vi "test1-LocalExternalStatusRegistration.vi"(8 "error in (no error)":errorcluster, 11 "TestCase in":refnum<class "testcase-CSMBroadcast.lvclass">) -> (0 "error out":errorcluster, 3 "TestCase out":refnum<class "testcase-CSMBroadcast.lvclass">)   [LabVIEW 2017, in "testcase-CSMBroadcast.lvclass"]
uses:
  testcase-CSMBroadcast.lvclass
  0b17d103-e67b-41be-a9eb-a2ee1311ff1f.vi
  5999693e-4f8a-4b34-ae87-f34dff5771be.vi
  de2dcf32-e0f3-4ce3-ae15-c78c2a65fbc0.vi
  52a2a10a-a04b-4bad-8df4-e1eb944f47cc.vi
  826f03dd-b4b5-4c6b-9085-8edf6da4f43b.vi
  src/user.lib/_NEVSTOP/Communicable State Machine(CSM)/AdvanceAPI/CSM - Revert Arguments-Safe String.vi
  src/user.lib/_NEVSTOP/Communicable State Machine(CSM)/_Shared/Trim Single-line Text.vi
  src/user.lib/_NEVSTOP/Communicable State Machine(CSM)/AdvanceAPI/CSM - Make String Arguments Safe.vi
  src/user.lib/_NEVSTOP/Communicable State Machine(CSM)/AdvanceAPI/CSM - Break Down Multiple States String.vi
  src/user.lib/_NEVSTOP/Communicable State Machine(CSM)/AdvanceAPI/CSM - Keywords.vi
  src/user.lib/_NEVSTOP/Communicable State Machine(CSM)/_Polymophic/CSM - Replace Marks in Messages.vi
  src/user.lib/_NEVSTOP/Communicable State Machine(CSM)/AdvanceAPI/CSM - Get Module Attribute.vi
  <vilib>/addons/_JKI Toolkits/VI Tester/TestCase.llb/TestCase.lvclass
  src/user.lib/_NEVSTOP/Communicable State Machine(CSM)/Communicable State Machine.lvlib
  C:/Program Files (x86)/National Instruments/LabVIEW 2017/vi.lib/addons/_JKI Toolkits/VI Tester/TestCase.llb/TestCase.lvclass
panel:
  out "One-Shot Unregistrations":string
  out "One-Shot Registrations":string
  out "LoopCount 2":i32
  out "State History":string
  out "LoopCount":i32
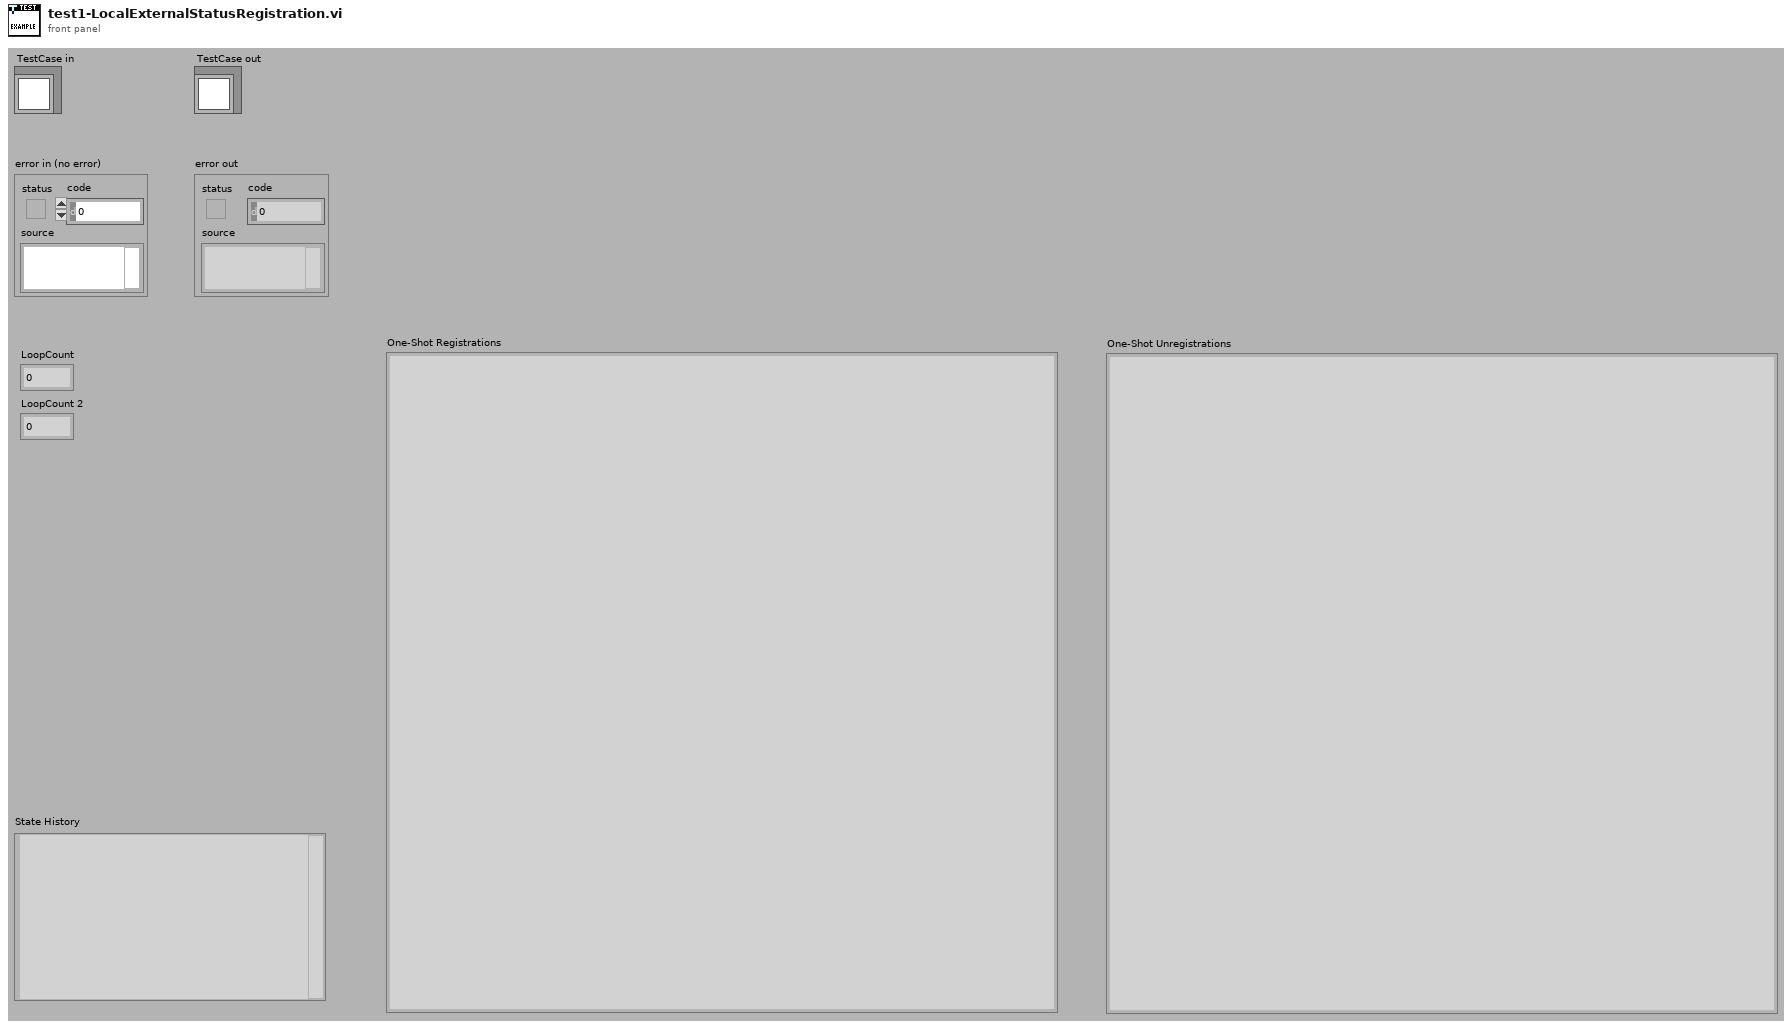
[diagram p1: front panel]
types:
  T1 = enum32{"Invalid", "Standard", "Closed", "Hidden", "Minimized", "Maximized"}
  T2 = enum32{"invalid app kind", "Development System", "Run Time System", "Student Edition", "Embedded LabVIEW", "Evaluation", "Custom"}
  T3 = typedef "Communicable State Machine.lvlib/_CSM_Response Source Message.ctl" = cluster{"‘State":string, "’Arguments":string, "’Error":errorcluster}
  T4 = cluster{"Current VI Reference":refnum<vi>, "Close Panel on Exit?":bool}
  T5 = cluster{"Core":cluster{"Current VI Reference":refnum<vi>, "Close Panel on Exit?":bool}, "Your Boolean data":bool, "Your string data":string}
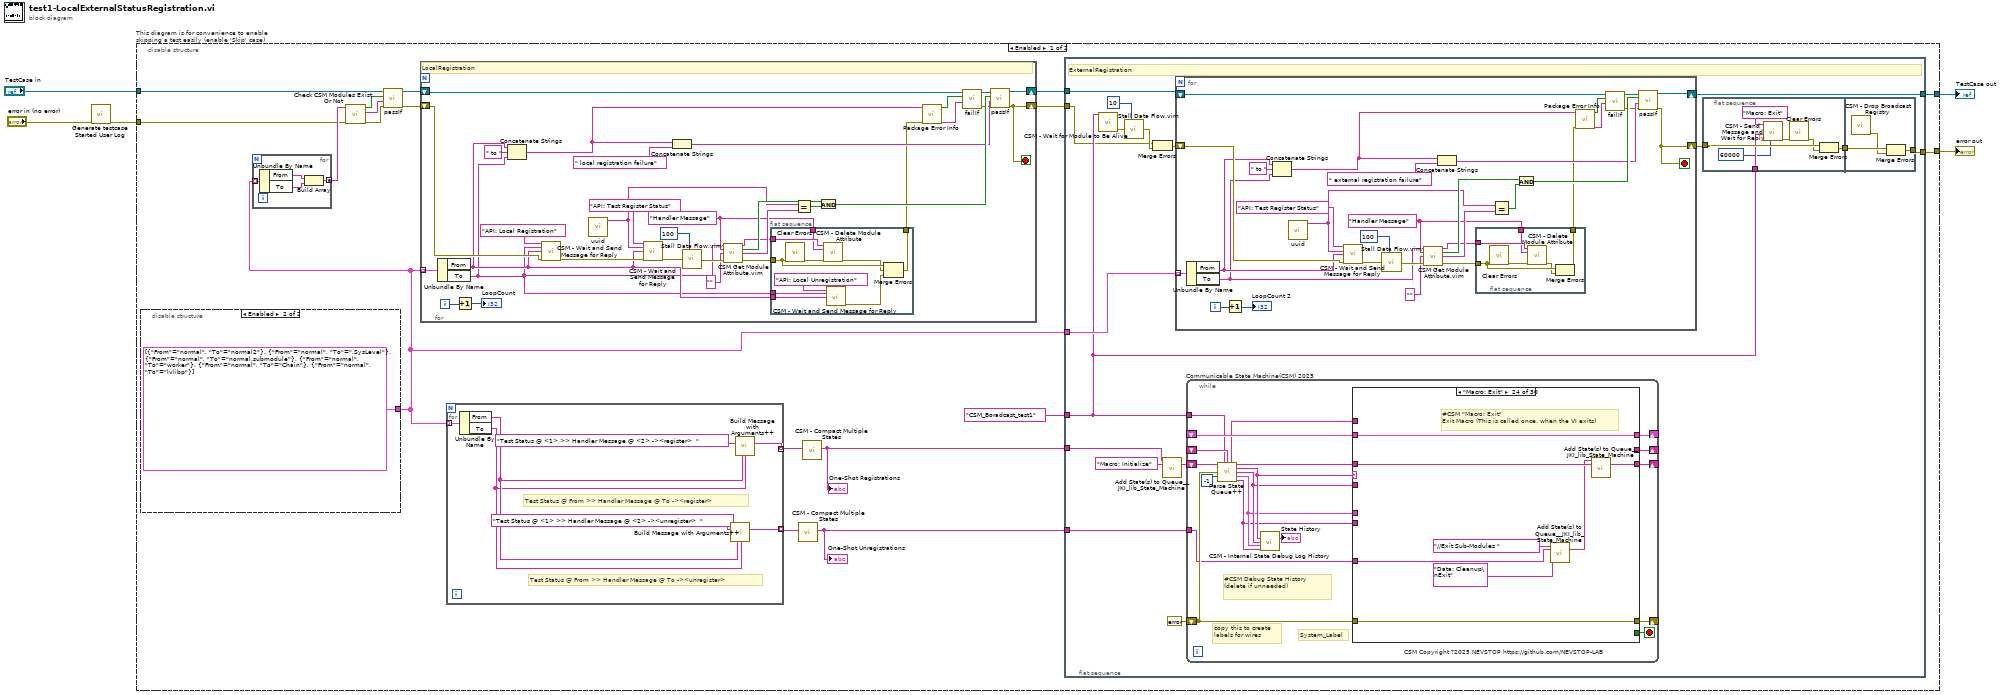
[diagram p0: block diagram]
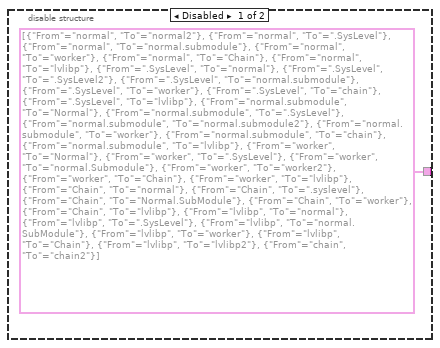
[diagram p2: hidden frame]
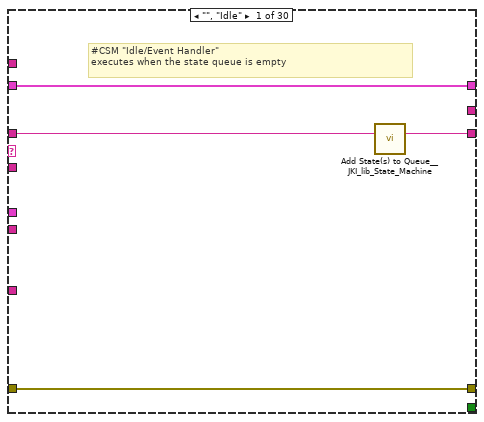
[diagram p3: hidden frame]
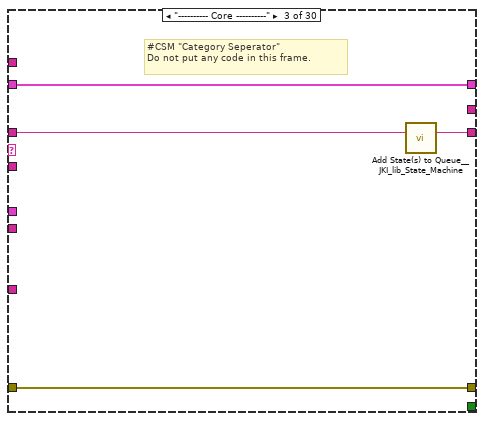
[diagram p5: hidden frame]
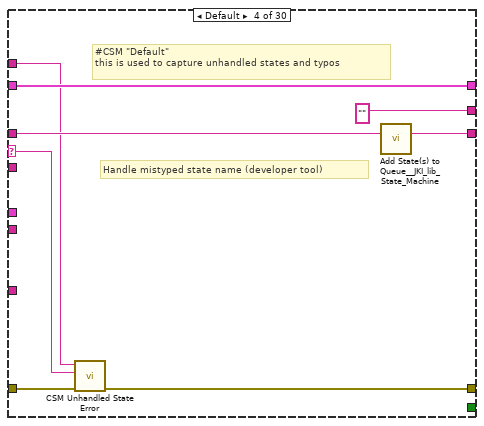
[diagram p6: hidden frame]
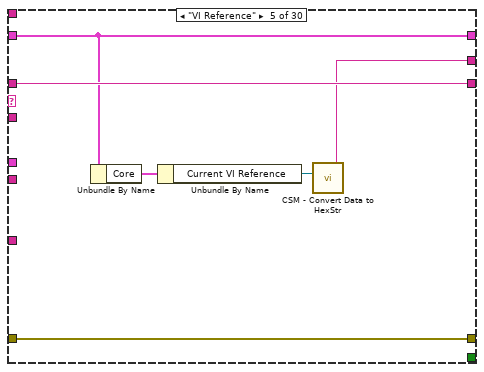
[diagram p7: hidden frame]
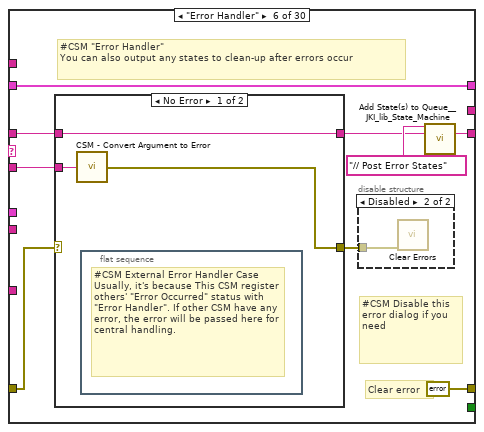
[diagram p8: hidden frame]
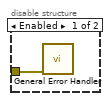
[diagram p9: hidden frame]
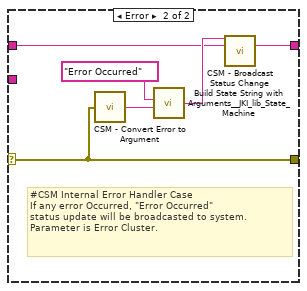
[diagram p10: hidden frame]
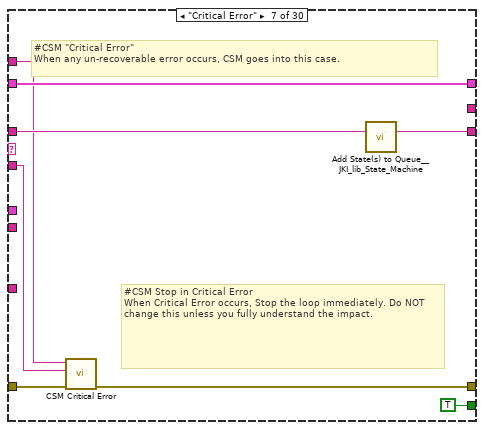
[diagram p11: hidden frame]
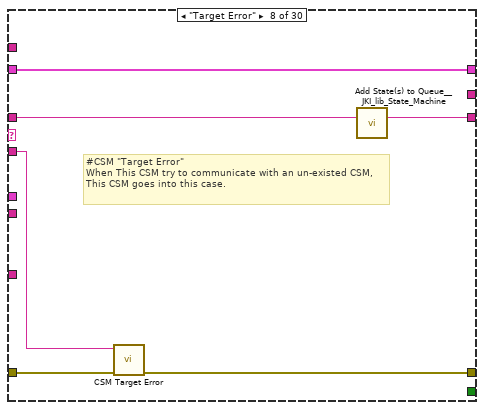
[diagram p12: hidden frame]
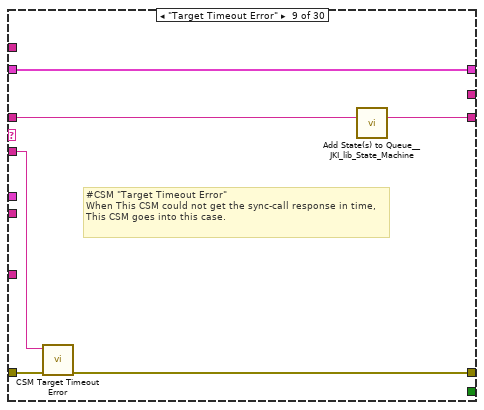
[diagram p13: hidden frame]
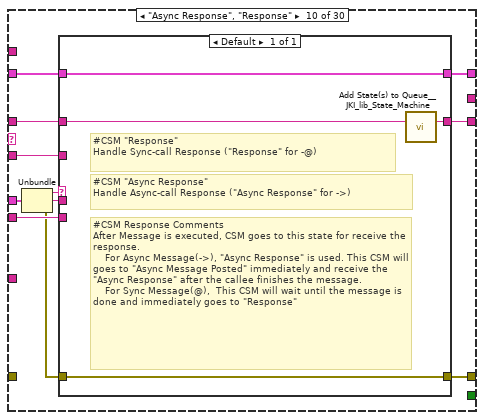
[diagram p14: hidden frame]
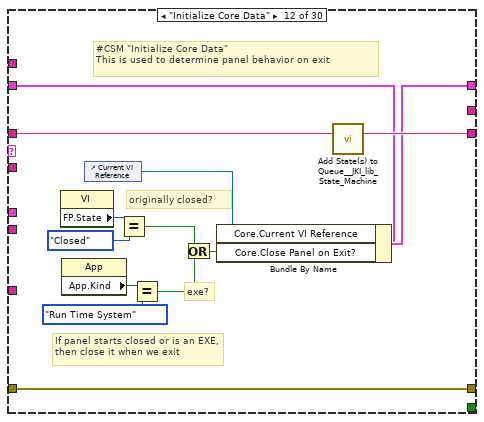
[diagram p16: hidden frame]
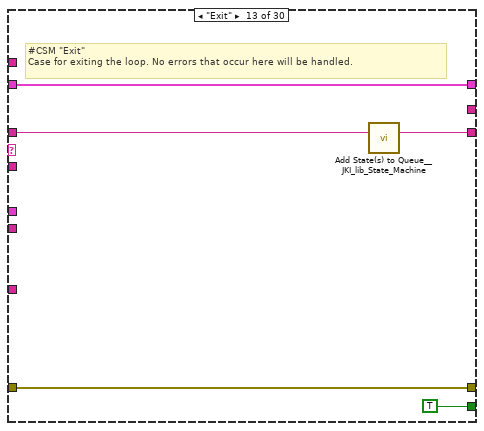
[diagram p17: hidden frame]
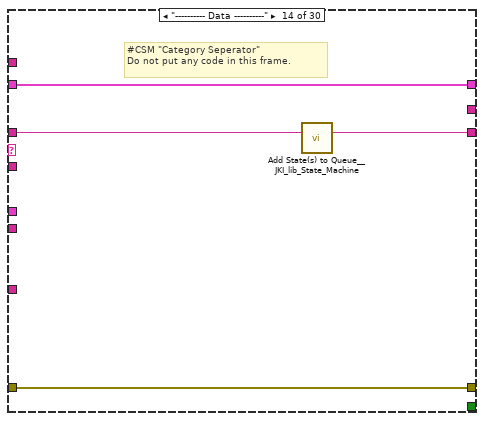
[diagram p18: hidden frame]
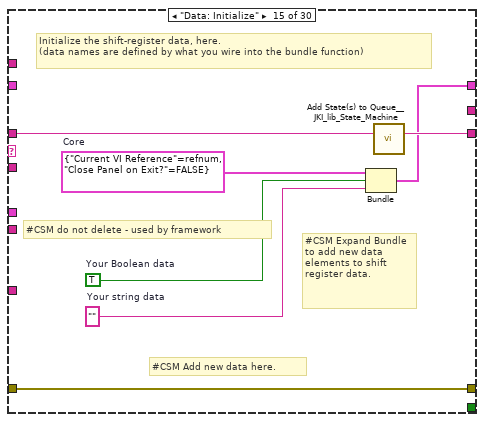
[diagram p19: hidden frame]
diagram:
  n1 = call "Generate testcase Started User Log.vi"("Error In"="error in (no error)") -> ("error out"=w1:errorcluster)  [unwired: 10 in]
  n2 = disable-structure "This diagram is for convenience to enable skipping a test easily (enable 'Skip' case)" shown="Enabled" {
    disable-tunnel: "TestCase in" -> [w11 w424]
    disable-tunnel: [w22 w422] -> w2
    disable-tunnel: [w16 w423] -> w4
    disable-tunnel: w1 -> [w9 w421]
    frame Enabled {
      n3 = disable-structure shown="Enabled" {
        disable-tunnel: [cluster{"From":string, "To":string}[] [{"From"="normal", "To"="normal2"}, {"From"="normal", "To"=".SysLevel"}, {"From"="normal", "To"="normal.submodule"}, {"From"="normal", "To"="worker"}, {"From"="normal", "To"="Chain"}, {"From"="normal", "To"="lvlibp"}, {"From"=".SysLevel", "To"="normal"}, {"From"=".SysLevel", "To"=".SysLevel2"}, {"From"=".SysLevel", "To"="normal.submodule"}, {"From"=".SysLevel", "To"="worker"}, {"From"=".SysLevel", "To"="chain"}, {"From"=".SysLevel", "To"="lvlibp"}, {"From"="normal.submodule", "To"="Normal"}, {"From"="normal.submodule", "To"=".SysLevel"}, {"From"="normal.submodule", "To"="normal.submodule2"}, {"From"="normal.submodule", "To"="worker"}, {"From"="normal.submodule", "To"="chain"}, {"From"="normal.submodule", "To"="lvlibp"}, {"From"="worker", "To"="Normal"}, {"From"="worker", "To"=".SysLevel"}, {"From"="worker", "To"="normal.Submodule"}, {"From"="worker", "To"="worker2"}, {"From"="worker", "To"="Chain"}, {"From"="worker", "To"="lvlibp"}, {"From"="Chain", "To"="normal"}, {"From"="Chain", "To"=".syslevel"}, {"From"="Chain", "To"="Normal.SubModule"}, {"From"="Chain", "To"="worker"}, {"From"="Chain", "To"="lvlibp"}, {"From"="lvlibp", "To"="normal"}, {"From"="lvlibp", "To"=".SysLevel"}, {"From"="lvlibp", "To"="normal.SubModule"}, {"From"="lvlibp", "To"="worker"}, {"From"="lvlibp", "To"="Chain"}, {"From"="lvlibp", "To"="lvlibp2"}, {"From"="chain", "To"="chain2"}] cluster{"From":string, "To":string}[] [{"From"="normal", "To"="normal2"}, {"From"="normal", "To"=".SysLevel"}, {"From"="normal", "To"="normal.submodule"}, {"From"="normal", "To"="worker"}, {"From"="normal", "To"="Chain"}, {"From"="normal", "To"="lvlibp"}]] -> w6
        frame Disabled {
        }
        frame Enabled {
        }
      }
      n4 = for {
        tunnel: w6 -> [w29] mode=indexing
        tunnel: [w26] -> w14 mode=concatenating
        n5 = Unbundle By Name(w29) -> ("From"=w28:string, "To"=w27:string)
        n6 = Build Array(w28, w27) -> (w26:string[])
      }
      n7 = call "Check CSM Modules Exist Or Not.vi"("error in"=w9, "CSM names in"=w14) -> ("error out"=w12:errorcluster, "Debug string"=w13:string, "All Modules Exist?"=w15:bool)  [unwired: 7 in]
      n8 = call-dynamic "passIf.vi"("error in (no error)"=w12, "message (\"\")"=w13, "pass"=w15, "TestCase in"=w11) -> ("error out"=w8:errorcluster, "TestCase out"=w10:refnum<class "testcase-CSMBroadcast.lvclass">)  [unwired: 6 in]
      n9 = for {
        shift-right: [w42] -> w21
        shift-left: w8 -> [w43]
        shift-right: [w49] -> w23
        shift-left: w10 -> [w34]
        tunnel: w6 -> [w60] mode=indexing
        i -> [w62]
        stop <- w42 stop-if-true
        w44 = "Handler Message" ("To")
        # "LocalRegistration"
        n10 = Unbundle By Name(w60) -> ("From"=w40:string, "To"=w39:string)
        n11 = Increment(x=w62) -> (x+1=→"LoopCount":i32)
        n12 = Concatenate Strings(w40, " to " ("string"), w39) -> (w30:string)
        n13 = call "CSM - Wait and Send Message for Reply.vi"("State"="API: Local Registration", "Arguments (\"\")"=w39, "Target Module"=w40, "Error In (No Error)"=w43) -> ("error out"=w57:errorcluster)  [unwired: 8 in, 3 out]
        n14 = call "uuid.vi"() -> ("UUID"=w51:string)  [unwired: 11 in]
        n15 = call "CSM - Wait and Send Message for Reply.vi"("State"="API: Test Register Status", "Arguments (\"\")"=w51, "Target Module"=w40, "Error In (No Error)"=w57) -> ("error out"=w56:errorcluster)  [unwired: 8 in, 3 out]
        n16 = Concatenate Strings(w30, " local registration failure" ("string")) -> (w37:string)
        n17 = call "Stall Data Flow.vim"("value in"=w56, "milliseconds to wait"=u32 100) -> ("value out"=w54:errorcluster)  [unwired: 1 out]
        n18 = call "CSM Get Module Attribute.vim"("CSM Name"=w39, "Attribute"=w44, "Default Value (Empty Variant)"="", "Error In"=w54) -> ("CSM Name (Dup)"=w45:string, "Found"=w53:bool, "Value"=w50:string, "error out"=w46:errorcluster)  [unwired: 7 in, 1 out]
        n19 = flat-sequence {
          tunnel: w46 -> [w66]
          tunnel: w45 -> [w71]
          tunnel: w44 -> [w70]
          tunnel: w39 -> [w68]
          tunnel: w40 -> [w67]
          tunnel: [w63] -> w31
          frame #0 {
            n20 = call <vilib>:"Clear Errors.vi"("error in (no error)"=w66) -> ("error out"=w72:errorcluster)  [unwired: 5 in, 1 out]
            n21 = call "CSM - Delete Module Attribute.vi"("CSM Name"=w71, "Attribute"=w70, "Error In"=w72) -> ("error out"=w65:errorcluster)  [unwired: 9 in, 3 out]
            n22 = call "CSM - Wait and Send Message for Reply.vi"("State"="API: Local Unregistration", "Arguments (\"\")"=w68, "Target Module"=w67) -> ("error out"=w64:errorcluster)  [unwired: 9 in, 3 out]
            n23 = Merge Errors(w66, w65, w64) -> (w63:errorcluster)
          }
        }
        n24 = Equal?(x=w51, y=w50) -> (x = y?=w48:bool)
        n25 = And(x=w53, y=w48) -> (x .and. y?=w47:bool)
        n26 = call "Package Error Info.vi"("error in"=w31, "String in"=w30) -> ("packed error info out"=w35:string, "error status"=w36:bool)  [unwired: 8 in]
        n27 = call-dynamic "failIf.vi"("message (\"\")"=w35, "fail"=w36, "TestCase in"=w34) -> ("error out"=w32:errorcluster, "TestCase out"=w33:refnum<class "testcase-CSMBroadcast.lvclass">)  [unwired: 7 in]
        n28 = call-dynamic "passIf.vi"("error in (no error)"=w32, "message (\"\")"=w37, "pass"=w47, "TestCase in"=w33) -> ("error out"=w42:errorcluster, "TestCase out"=w49:refnum<class "testcase-CSMBroadcast.lvclass">)  [unwired: 6 in]
      }
      n29 = for {
        tunnel: w6 -> [w78] mode=indexing
        tunnel: [w77] -> w20 mode=indexing
        tunnel: [w73] -> w18 mode=indexing
        # "Test Status @ From >> Handler Message @ To -><unregister>"
        # "Test Status @ From >> Handler Message @ To -><register>"
        n30 = Unbundle By Name(w78) -> ("From"=w75:string, "To"=w74:string)
        n31 = call-poly "Build Message with Arguments++.vi"("States With Replace Token"="Test Status @ <1> >> Handler Message @ <2> -><unregister>  " ("State"), "<1>"=w75, "<2>"=w74) -> ("States"=w73:string)  [unwired: 12 in]
        n32 = call-poly "Build Message with Arguments++.vi"("States With Replace Token"="Test Status @ <1> >> Handler Message @ <2> -><register>  " ("State"), "<1>"=w75, "<2>"=w74) -> ("States"=w77:string)  [unwired: 12 in]
      }
      n33 = call "CSM - Compact Multiple States.vi"("Multiple States"=w18) -> ("States"=w17:string)  [unwired: 9 in]
      "One-Shot Unregistrations" <- w17
      n34 = call "CSM - Compact Multiple States.vi"("Multiple States"=w20) -> ("States"=w19:string)  [unwired: 9 in]
      "One-Shot Registrations" <- w19
      n35 = flat-sequence {
        tunnel: w23 -> [w93]
        tunnel: [w92] -> w22
        tunnel: w21 -> [w80]
        tunnel: w6 -> [w91]
        tunnel: w19 -> [w90]
        tunnel: w17 -> [w87]
        tunnel: [w85] -> w16
        tunnel: "CSM_Boradcast_test1" ("Name (\"\" to Use UUID)") -> [w84]
        frame #0 {
          # "ExternalRegistration"
          n36 = call "CSM - Wait for Module to Be Alive.vi"("CSM Name"=w84) -> ("error out"=w83:errorcluster)  [unwired: 12 in, 2 out]
          n37 = call "Stall Data Flow.vim"("value in"=w83, "milliseconds to wait"=u32 10) -> ("value out"=w82:errorcluster)  [unwired: 1 out]
          n38 = Merge Errors(w80, w82) -> (w88:errorcluster)
          n39 = call <vilib>:"Add State(s) to Queue__JKI_lib_State_Machine.vi"("State(s) in Front (\"\")"=w90, "State(s) in (\"\")"="Macro: Initialize" ("Init State(\"Macro: Initialize\")")) -> ("States Out"=w94:string)  [unwired: 13 in]
          n40 = for {
            shift-right: [w119] -> w89
            shift-left: w88 -> [w120]
            shift-right: [w126] -> w92
            shift-left: w93 -> [w111]
            tunnel: w91 -> [w135] mode=indexing
            i -> [w137]
            stop <- w119 stop-if-true
            w121 = "Handler Message" ("To")
            n41 = Unbundle By Name(w135) -> ("From"=w116:string, "To"=w115:string)
            n42 = Increment(x=w137) -> (x+1=→"LoopCount 2":i32)
            n43 = Concatenate Strings(w116, " to " ("string"), w115) -> (w107:string)
            n44 = call "uuid.vi"() -> ("UUID"=w128:string)  [unwired: 11 in]
            n45 = call "CSM - Wait and Send Message for Reply.vi"("State"="API: Test Register Status", "Arguments (\"\")"=w128, "Target Module"=w116, "Error In (No Error)"=w120) -> ("error out"=w133:errorcluster)  [unwired: 8 in, 3 out]
            n46 = call "Stall Data Flow.vim"("value in"=w133, "milliseconds to wait"=u32 100) -> ("value out"=w131:errorcluster)  [unwired: 1 out]
            n47 = call "CSM Get Module Attribute.vim"("CSM Name"=w115, "Attribute"=w121, "Default Value (Empty Variant)"="", "Error In"=w131) -> ("CSM Name (Dup)"=w122:string, "Found"=w130:bool, "Value"=w127:string, "error out"=w123:errorcluster)  [unwired: 7 in, 1 out]
            n48 = Concatenate Strings(w107, " external registration failure" ("string")) -> (w114:string)
            n49 = flat-sequence {
              tunnel: w123 -> [w140]
              tunnel: w122 -> [w142]
              tunnel: w121 -> [w141]
              tunnel: [w138] -> w108
              frame #0 {
                n50 = call <vilib>:"Clear Errors.vi"("error in (no error)"=w140) -> ("error out"=w143:errorcluster)  [unwired: 5 in, 1 out]
                n51 = call "CSM - Delete Module Attribute.vi"("CSM Name"=w142, "Attribute"=w141, "Error In"=w143) -> ("error out"=w139:errorcluster)  [unwired: 9 in, 3 out]
                n52 = Merge Errors(w140, w139) -> (w138:errorcluster)
              }
            }
            n53 = Equal?(x=w128, y=w127) -> (x = y?=w125:bool)
            n54 = And(x=w130, y=w125) -> (x .and. y?=w124:bool)
            n55 = call "Package Error Info.vi"("error in"=w108, "String in"=w107) -> ("packed error info out"=w112:string, "error status"=w113:bool)  [unwired: 8 in]
            n56 = call-dynamic "failIf.vi"("message (\"\")"=w112, "fail"=w113, "TestCase in"=w111) -> ("error out"=w109:errorcluster, "TestCase out"=w110:refnum<class "testcase-CSMBroadcast.lvclass">)  [unwired: 7 in]
            n57 = call-dynamic "passIf.vi"("error in (no error)"=w109, "message (\"\")"=w114, "pass"=w124, "TestCase in"=w110) -> ("error out"=w119:errorcluster, "TestCase out"=w126:refnum<class "testcase-CSMBroadcast.lvclass">)  [unwired: 6 in]
          }
          n58 = while "Communicable State Machine(CSM) 2025" {
            shift-right: [w157] -> _
            shift-left: _ -> [w156]
            shift-right: [w160] -> _
            shift-left: errorcluster {"status"=FALSE, "code"=0, "source"=""} ("error out") -> [w155]
            shift-right: [w159] -> _
            shift-left: w94 -> [w161]
            shift-right: [w154] -> _
            shift-left: _ -> [w148]
            tunnel: w87 -> [w145]
            tunnel: w84 -> [w144]
            stop <- w158 stop-if-true
            # "#CSM Debug State History\n(delete if unneeded)"
            # "copy this to create labels for wires"
            # "System_Label"
            # "CSM Copyright ?2025 NEVSTOP https://github.com/NEVSTOP-LAB"
            n59 = call "Parse State Queue++.vi"("State Queue"=w161, "Name (\"\" to Use UUID)"=w144, "Response Arguments"=w148, "Previous Error"=w155, "Dequeue (1 ms)"=-1 ("Timeout")) -> ("Name Used"=w149:string, "Remaining States"=w162:string, "Current State"=w153:string, "Arguments"=w152:string, "Additional Information"=w151:T3, "Source CSM"=w150:string)  [unwired: 5 in]
            n60 = call "CSM - Internal State Debug Log History.vi"("State"=w153, "Arguments (\"\")"=w152, ">> Response Source Message >>"=w151, "Source (\"\")"=w150) -> ("Debug Log"=→"State History":string)  [unwired: 11 in]
            n61 = case shown="\"Macro: Exit\"" w153 {
              selector: w153 -> [_ _ _ w176 _ _ _ _ _ _ _ _ _ _ _ _ _ _ _ _ _ _ _ _ _ _ _ _ _ _]
              tunnel: w162 -> [w163 w168 w173 w180 w186 w192 w213 w219 w225 w233 w244 w258 w263 w267 w274 w276 w283 w287 w291 w297 w312 w381 w386 w394 w396 w400 w405 w412 w416 w420]
              tunnel: w152 -> [_ _ _ _ _ w191 w209 w218 w223 w232 _ _ _ _ _ _ _ _ _ w292 w306 _ _ _ _ _ w403 _ _ _]
              tunnel: w156 -> [w164 w167 w170 w178 w185 w195 w214 w220 w226 w235 w243 w251 w261 w264 _ w275 w278 w284 w289 w295 w308 w378 w383 w391 w395 w399 w404 w409 w413 w417]
              tunnel: [w165 w169 w171 w174 w187 errorcluster {"status"=FALSE, "code"=0, "source"=""} ("error out") w210 w216 w222 w238 w245 w255 w260 w265 w271 w277 w279 w285 w288 w293 w309 w379 w384 w392 w397 w401 w406 w410 w414 w418] -> w160
              tunnel: w155 -> [w165 w169 w171 w181 w187 w193 w215 w217 w224 _ w245 w255 w260 w265 w271 w277 w280 w285 w288 w294 w310 w379 w384 w392 w397 w401 w406 w410 w414 w418]
              tunnel: [w166 w168 w172 w179 w186 w188 w212 w221 w227 w234 w244 w257 w262 w266 w273 w276 w282 w286 w290 w296 w311 w380 w385 w393 w396 w400 w405 w411 w415 w419] -> w159
              tunnel: [_ _ _ _ _ _ TRUE _ _ _ _ _ TRUE _ _ _ _ _ _ _ _ _ _ _ _ _ _ _ _ _] -> w158
              tunnel: [w164 w167 w170 w178 w185 w195 w214 w220 w226 w236 w243 w256 w261 w264 w272 w275 w278 w284 w289 w295 w308 w378 w383 w391 w395 w399 w404 w409 w413 w417] -> w157
              tunnel: w150 -> [_ _ _ _ _ _ _ _ _ w230 _ _ _ _ _ _ _ _ _ _ _ _ _ _ _ _ _ _ _ _]
              tunnel: w151 -> [_ _ _ _ _ _ _ _ _ w237 _ _ _ _ _ _ _ _ _ _ _ _ _ _ _ _ _ _ _ _]
              tunnel: [_ _ _ "" w182 _ _ _ _ _ _ _ _ _ _ _ _ _ _ _ _ _ _ _ _ "API1 Response" w402 _ _ _] -> w154
              tunnel: w149 -> [_ _ _ w175 _ _ w208 _ _ _ _ _ _ _ _ _ _ _ _ _ _ _ _ _ _ _ _ _ _ _]
              tunnel: w145 -> [_ _ _ _ _ _ _ _ _ _ _ _ _ _ _ _ _ _ _ _ _ _ _ w387 _ _ _ _ _ _]
              frame "", "Idle" {
                # "#CSM \"Idle/Event Handler\"\nexecutes when the state queue is empty"
                n62 = call <vilib>:"Add State(s) to Queue__JKI_lib_State_Machine.vi"("State(s) in (\"\")"=w163) -> ("States Out"=w166:string)  [unwired: 14 in]
              }
              frame "CSM Documentation" {
                # "#CSM README FIRST\n\nCommunicable State Machine(CSM) is a LabVIEW application framework that builds upon JKI State Machine(JKISM). It follows the pattern of JKISM and extends the keywords to describe message communication between modules, including concepts such as Sync-Message, Async-Message, Subscription/Unsubscription of status - essential elements for creating reusable code modules. For more information, please visit the CSM wiki: https://nevstop-lab.github.io/CSM-Wiki/\n\nFor instructions on JKI State Machine, visit: http://jki.net/state-machine/\nFor information about CSM, visit: https://github.com/NEVSTOP-LAB"
                # "#CSM \"Documentation\"\nCase for holding CSM Documenation"
              }
              frame "---------- Core ----------" {
                # "#CSM \"Category Seperator\"\nDo not put any code in this frame."
                n63 = call <vilib>:"Add State(s) to Queue__JKI_lib_State_Machine.vi"("State(s) in (\"\")"=w173) -> ("States Out"=w172:string)  [unwired: 14 in]
              }
              frame Default {
                # "#CSM \"Default\"\nthis is used to capture unhandled states and typos"
                # "Handle mistyped state name (developer tool)"
                n64 = call "CSM Unhandled State Error.vi"("error in (no error)"=w181, "Undefined State"=w176, "CSM Name"=w175) -> ("error out"=w174:errorcluster)  [unwired: 8 in]
                n65 = call <vilib>:"Add State(s) to Queue__JKI_lib_State_Machine.vi"("State(s) in (\"\")"=w180) -> ("States Out"=w179:string)  [unwired: 14 in]
              }
              frame "VI Reference" {
                n66 = Unbundle By Name(w185) -> ("Core"=w184:T4)
                n67 = Unbundle By Name(w184) -> ("Current VI Reference"=w183:refnum<vi>)
                n68 = call "CSM - Convert Data to HexStr.vi"("Variant"=w183) -> ("HEX String (0-9,A-F)"=w182:string)  [unwired: 8 in]
              }
              frame "Error Handler" {
                # "#CSM Disable this error dialog if you need"
                # "#CSM \"Error Handler\"\nYou can also output any states to clean-up after errors occur"
                # "Clear error"
                n69 = case shown="No Error" w193 {
                  selector: w193 -> [_ w202]
                  tunnel: [w201 w204] -> w189
                  tunnel: w192 -> [w201 w203]
                  tunnel: w191 -> [w200 _]
                  tunnel: [w199 w202] -> w194
                  frame No Error {
                    n70 = call "CSM - Convert Argument to Error.vi"("Argument"=w200) -> ("Error"=w199:errorcluster)  [unwired: 4 in]
                    n71 = flat-sequence {
                      frame #0 {
                        # "#CSM External Error Handler Case\nUsually, it's because This CSM register others' \"Error Occurred\" status with \"Error Handler\". If other CSM have any error, the error will be passed here for central handling."
                      }
                    }
                  }
                  frame Error {
                    # "#CSM Internal Error Handler Case \nIf any error Occurred, \"Error Occurred\" \nstatus update will be broadcasted to system.\nParameter is Error Cluster."
                    n72 = call "CSM - Convert Error to Argument.vi"("Error"=w202) -> ("Argument"=w206:string)  [unwired: 4 in]
                    n73 = call <vilib>:"Build State String with Arguments__JKI_lib_State_Machine.vi"("Arguments (\"\")"=w206, "State"="Error Occurred" ("Status with Arguments")) -> ("State with Arguments"=w205:string)  [unwired: 4 in]
                    n74 = call "CSM - Broadcast Status Change.vi"("Status With Arguments"=w205, "State Queue"=w203) -> ("Remaining States"=w204:string)  [unwired: 13 in]
                  }
                }
                n75 = disable-structure shown="Disabled" {
                  disable-tunnel: w194 -> [w197 w198]
                  frame Enabled {
                    n76 = call <vilib>:"General Error Handler.vi"("error in (no error)"=w197) -> ()  [unwired: 10 in, 5 out]
                  }
                  frame Disabled {
                    n77 = call <vilib>:"Clear Errors.vi"("error in (no error)"=w198) -> ()  [unwired: 5 in, 2 out]
                  }
                }
                n78 = call <vilib>:"Add State(s) to Queue__JKI_lib_State_Machine.vi"("State(s) in Front (\"\")"="// Post Error States", "State(s) in (\"\")"=w189) -> ("States Out"=w188:string)  [unwired: 13 in]
              }
              frame "Critical Error" {
                # "#CSM Stop in Critical Error\nWhen Critical Error occurs, Stop the loop immediately. Do NOT change this unless you fully understand the impact."
                # "#CSM \"Critical Error\"\nWhen any un-recoverable error occurs, CSM goes into this case."
                n79 = call "CSM Critical Error.vi"("error in (no error)"=w215, "Arugments (As Reason)"=w209, "CSM Name"=w208) -> ("error out"=w210:errorcluster)  [unwired: 8 in]
                n80 = call <vilib>:"Add State(s) to Queue__JKI_lib_State_Machine.vi"("State(s) in (\"\")"=w213) -> ("States Out"=w212:string)  [unwired: 14 in]
              }
              frame "Target Error" {
                # "#CSM \"Target Error\"\nWhen This CSM try to communicate with an un-existed CSM, This CSM goes into this case."
                n81 = call "CSM Target Error.vi"("error in (no error)"=w217, "Arguments (As CSM Name)"=w218) -> ("error out"=w216:errorcluster)  [unwired: 9 in]
                n82 = call <vilib>:"Add State(s) to Queue__JKI_lib_State_Machine.vi"("State(s) in (\"\")"=w219) -> ("States Out"=w221:string)  [unwired: 14 in]
              }
              frame "Target Timeout Error" {
                # "#CSM \"Target Timeout Error\"\nWhen This CSM could not get the sync-call response in time, This CSM goes into this case."
                n83 = call "CSM Target Timeout Error.vi"("error in (no error)"=w224, "Arguments (As CSM Name)"=w223) -> ("error out"=w222:errorcluster)  [unwired: 9 in]
                n84 = call <vilib>:"Add State(s) to Queue__JKI_lib_State_Machine.vi"("State(s) in (\"\")"=w225) -> ("States Out"=w227:string)  [unwired: 14 in]
              }
              frame "Async Response", "Response" {
                n85 = Unbundle(w237) -> ("‘State"=w231:string, "’Arguments"=w229:string, "’Error"=w228:errorcluster)
                n86 = case shown="Default" w231 {
                  tunnel: [w242] -> w238
                  tunnel: w228 -> [w242]
                  tunnel: [w241] -> w236
                  tunnel: w235 -> [w241]
                  tunnel: [w239] -> w234
                  tunnel: w233 -> [w240]
                  tunnel: w232 -> [_]
                  tunnel: w230 -> [_]
                  tunnel: w229 -> [_]
                  frame Default {
                    # "#CSM Response Comments\nAfter Message is executed, CSM goes to this state for receive the response.\n    For Async Message(->), \"Async Response\" is used. This CSM will goes to \"Async Message Posted\" immediately and receive the \"Async Response\" after the callee finishes the message.\n    For Sync Message(@),  This CSM will wait until the message is done and immediately goes to \"Response\""
                    # "#CSM \"Async Response\"\nHandle Async-call Response (\"Async Response\" for ->)"
                    # "#CSM \"Response\"\nHandle Sync-call Response (\"Response\" for -@)"
                    n87 = call <vilib>:"Add State(s) to Queue__JKI_lib_State_Machine.vi"("State(s) in (\"\")"=w240) -> ("States Out"=w239:string)  [unwired: 14 in]
                  }
                }
              }
              frame "Async Message Posted" {
                # "#CSM \"Async Message Posted\"\nAfter Async Message is posted (-> or ->| ), CSM goes to this state for post-action.\nYou can use Argument - State to tell which Async Message is called."
              }
              frame "Initialize Core Data" {
                # "#CSM \"Initialize Core Data\"\nThis is used to determine panel behavior on exit"
                # "originally closed?"
                # "exe?"
                # "If panel starts closed or is an EXE, then close it when we exit"
                n88 = property class="VI"() -> ("FP.State"=w248:T1)  [unwired: 2 in, 2 out]
                n89 = property class="App"() -> ("App.Kind"=w254:T2)  [unwired: 2 in, 2 out]
                n90 = control-ref of="Current VI Reference"() -> (w249:refnum<vi>)
                n91 = Equal?(x=w248, y=T1."Closed" ("Front Panel Window:State")) -> (x = y?=w246:bool)
                n92 = Equal?(x=w254, y=T2."Run Time System" ("Application:Kind")) -> (x = y?=w252:bool)
                n93 = Or(x=w246, y=w252) -> (x .or. y?=w250:bool)
                n94 = Bundle By Name(cluster=w251, "Core.Current VI Reference"=w249, "Core.Close Panel on Exit?"=w250) -> (w256:T5)
                n95 = call <vilib>:"Add State(s) to Queue__JKI_lib_State_Machine.vi"("State(s) in (\"\")"=w258) -> ("States Out"=w257:string)  [unwired: 14 in]
              }
              frame "Exit" {
                # "#CSM \"Exit\"\nCase for exiting the loop. No errors that occur here will be handled."
                n96 = call <vilib>:"Add State(s) to Queue__JKI_lib_State_Machine.vi"("State(s) in (\"\")"=w263) -> ("States Out"=w262:string)  [unwired: 14 in]
              }
              frame "---------- Data ----------" {
                # "#CSM \"Category Seperator\"\nDo not put any code in this frame."
                n97 = call <vilib>:"Add State(s) to Queue__JKI_lib_State_Machine.vi"("State(s) in (\"\")"=w267) -> ("States Out"=w266:string)  [unwired: 14 in]
              }
              frame "Data: Initialize" {
                w268 = T4 {"Current VI Reference"=refnum, "Close Panel on Exit?"=FALSE}  # Core
                w270 = TRUE  # Your Boolean data
                w269 = ""  # Your string data
                # "#CSM do not delete - used by framework"
                # "#CSM Expand Bundle to add new data elements to shift register data."
                # "#CSM Add new data here."
                # "Initialize the shift-register data, here.\n(data names are defined by what you wire into the bundle function)"
                n98 = Bundle("Core"=w268, "Your Boolean data"=w270, "Your string data"=w269) -> (w272:T5)  [unwired: 1 in]
                n99 = call <vilib>:"Add State(s) to Queue__JKI_lib_State_Machine.vi"("State(s) in (\"\")"=w274) -> ("States Out"=w273:string)  [unwired: 14 in]
              }
              frame "Data: Update Indicators" {
              }
              frame "Data: Cleanup" {
                # "Cleanup any data and references, here.\n(this is called automatically, by the Macro: Exit)"
                n100 = Unbundle By Name(w278) -> ("Core.Current VI Reference"=w281:refnum<vi>)
                n101 = Close Reference(reference=w281, error in (no error)=w280) -> (error out=w279:errorcluster)
                n102 = call <vilib>:"Add State(s) to Queue__JKI_lib_State_Machine.vi"("State(s) in (\"\")"=w283) -> ("States Out"=w282:string)  [unwired: 14 in]
              }
              frame "---------- UI ----------" {
                # "#CSM \"Category Seperator\"\nDo not put any code in this frame."
                n103 = call <vilib>:"Add State(s) to Queue__JKI_lib_State_Machine.vi"("State(s) in (\"\")"=w287) -> ("States Out"=w286:string)  [unwired: 14 in]
              }
              frame "UI: Initialize" {
                # "#CSM \"UI: Initialize\"\nInitialize the User Interface, here.\n(this is called automatically, by the Macro: Init)"
                n104 = call <vilib>:"Add State(s) to Queue__JKI_lib_State_Machine.vi"("State(s) in (\"\")"=w291) -> ("States Out"=w290:string)  [unwired: 14 in]
              }
              frame "UI: Cursor Set" {
                # "#CSM \"UI: Cursor Set\"\nSet and Unset Cursor Busy.\n(Usage: \"UI: Cursor Set >> Busy|Idle\")"
                # "Argument"
                n105 = disable-structure shown="TARGET_TYPE!=Windows" {
                  disable-tunnel: w294 -> [w300 w305]
                  disable-tunnel: [w299 w305] -> w293
                  disable-tunnel: w292 -> [w298 _]
                  frame condition #0 (active) {
                    n106 = case shown="\"Idle\", Default" w298 {
                      tunnel: w300 -> [w302 w304]
                      tunnel: [w301 w303] -> w299
                      frame "Idle", Default {
                        n107 = call <vilib>:"Unset Busy.vi"("error in (no error)"=w302) -> ("error out"=w301:errorcluster)  [unwired: 10 in]
                      }
                      frame "Busy" {
                        n108 = call <vilib>:"Set Busy.vi"("error in (no error)"=w304) -> ("error out"=w303:errorcluster)  [unwired: 9 in, 1 out]
                      }
                    }
                  }
                  frame condition #1 {
                  }
                }
                n109 = call <vilib>:"Add State(s) to Queue__JKI_lib_State_Machine.vi"("State(s) in (\"\")"=w297) -> ("States Out"=w296:string)  [unwired: 14 in]
              }
              frame "UI: Front Panel State" {
                # "#CSM \"UI: Front Panel State\"\nSet Front Panel Open or Closed\n(Usage: \"UI: Front Panel State >> Open|Close\")"
                # "Argument"
                n110 = Unbundle By Name(w308) -> ("Core.Current VI Reference"=w307:refnum<vi>)
                n111 = call <vilib>:"Add State(s) to Queue__JKI_lib_State_Machine.vi"("State(s) in (\"\")"=w312) -> ("States Out"=w311:string)  [unwired: 14 in]
                n112 = case shown="\"Close\", \"Closed\"" w306 {
                  tunnel: w310 -> [w318 w333 w344 w357 w370]
                  tunnel: [w320 w334 w346 w359 w372] -> w309
                  tunnel: w307 -> [w319 w331 w345 w358 w371]
                  frame "Open", "Standard", Default {
                    w313 = T1."Standard" ("State")
                    n113 = property class="VI"(reference=w319, error in=w318) -> (reference out=w316:refnum<vi>, error out=w317:errorcluster, "FP.State"=w315:T1)
                    n114 = Not Equal?(x=w315, y=w313) -> (x != y?=w314:bool)
                    n115 = case shown="True" w314 {
                      tunnel: [w324 w326] -> w320
                      tunnel: w317 -> [w323 w326]
                      tunnel: w316 -> [w322 _]
                      tunnel: w313 -> [w321 _]
                      frame True {
                        n116 = invoke class="VI" method="FP.Open"(reference=w322, error in=w323, "Activate"=TRUE, "State"=w321) -> (error out=w324:errorcluster)  [unwired: 1 in, 4 out]
                      }
                      frame False {
                      }
                    }
                  }
                  frame "Close", "Closed" {
                    n117 = property class="VI"(reference=w331, error in=w333) -> (reference out=w330:refnum<vi>, error out=w332:errorcluster, "FP.State"=w328:T1)
                    n118 = Not Equal?(x=w328, y=T1."Closed" ("Front Panel Window:State")) -> (x != y?=w327:bool)
                    n119 = case shown="False" w327 {
                      tunnel: [w335 w338] -> w334
                      tunnel: w332 -> [w335 w337]
                      tunnel: w330 -> [_ w336]
                      frame False {
                      }
                      frame True {
                        n120 = invoke class="VI" method="FP.Close"(reference=w336, error in=w337) -> (error out=w338:errorcluster)  [unwired: 1 in, 2 out]
                      }
                    }
                  }
                  frame "Hidden", "Hide" {
                    w339 = T1."Hidden" ("State")
                    n121 = property class="VI"(reference=w345, error in=w344) -> (reference out=w342:refnum<vi>, error out=w343:errorcluster, "FP.State"=w341:T1)
                    n122 = Not Equal?(x=w341, y=w339) -> (x != y?=w340:bool)
                    n123 = case shown="True" w340 {
                      tunnel: [w350 w351] -> w346
                      tunnel: w343 -> [w349 w351]
                      tunnel: w342 -> [w348 _]
                      tunnel: w339 -> [w347 _]
                      frame True {
                        n124 = invoke class="VI" method="FP.Open"(reference=w348, error in=w349, "State"=w347) -> (error out=w350:errorcluster)  [unwired: 2 in, 4 out]
                      }
                      frame False {
                      }
                    }
                  }
                  frame "Minimize", "Minimized" {
                    w352 = T1."Minimized" ("State")
                    n125 = property class="VI"(reference=w358, error in=w357) -> (reference out=w355:refnum<vi>, error out=w356:errorcluster, "FP.State"=w354:T1)
                    n126 = Not Equal?(x=w354, y=w352) -> (x != y?=w353:bool)
                    n127 = case shown="True" w353 {
                      tunnel: [w363 w364] -> w359
                      tunnel: w356 -> [w362 w364]
                      tunnel: w355 -> [w361 _]
                      tunnel: w352 -> [w360 _]
                      frame True {
                        n128 = invoke class="VI" method="FP.Open"(reference=w361, error in=w362, "State"=w360) -> (error out=w363:errorcluster)  [unwired: 2 in, 4 out]
                      }
                      frame False {
                      }
                    }
                  }
                  frame "Maximize", "Maximized" {
                    w365 = T1."Maximized" ("State")
                    n129 = property class="VI"(reference=w371, error in=w370) -> (reference out=w368:refnum<vi>, error out=w369:errorcluster, "FP.State"=w367:T1)
                    n130 = Not Equal?(x=w367, y=w365) -> (x != y?=w366:bool)
                    n131 = case shown="True" w366 {
                      tunnel: [w376 w377] -> w372
                      tunnel: w369 -> [w375 w377]
                      tunnel: w368 -> [w374 _]
                      tunnel: w365 -> [w373 _]
                      frame True {
                        n132 = invoke class="VI" method="FP.Open"(reference=w374, error in=w375, "State"=w373) -> (error out=w376:errorcluster)  [unwired: 2 in, 4 out]
                      }
                      frame False {
                      }
                    }
                  }
                }
              }
              frame "---------- Macro ----------" {
                # "#CSM \"Category Seperator\"\nDo not put any code in this frame."
                n133 = call <vilib>:"Add State(s) to Queue__JKI_lib_State_Machine.vi"("State(s) in (\"\")"=w381) -> ("States Out"=w380:string)  [unwired: 14 in]
              }
              frame "Macro: Initialize" {
                # "#CSM \"Macro: Initialize\"\nInitialization Macro (This is called once, when the VI starts)"
                n134 = call <vilib>:"Add State(s) to Queue__JKI_lib_State_Machine.vi"("State(s) in Front (\"\")"="Data: Initialize\nInitialize Core Data\nData: Update Indicators", "State(s) in (\"\")"=w386) -> ("States Out"=w385:string)  [unwired: 13 in]
              }
              frame "Macro: Exit" {
                # "#CSM \"Macro: Exit\"\nExit Macro (This is called once, when the VI exits)"
                n135 = call <vilib>:"Add State(s) to Queue__JKI_lib_State_Machine.vi"("State(s) in Front (\"\")"="//Exit Sub-Modules ", "State(s) in (\"\")"=w387, "State(s) at Back (\"\")"="Data: Cleanup\nExit") -> ("States Out"=w389:string)  [unwired: 12 in]
                n136 = call <vilib>:"Add State(s) to Queue__JKI_lib_State_Machine.vi"("State(s) in Front (\"\")"=w389, "State(s) in (\"\")"=w394) -> ("States Out"=w393:string)  [unwired: 13 in]
              }
              frame "---------- API ----------" {
                # "#CSM \"Category Seperator\"\nDo not put any code in this frame."
              }
              frame "API: API1" {
                # "#CSM API Example\nCopy/Rename this case for your own API"
                # "#CSM Response\nConnect this to return the response of your API"
                # "#CSM >> Msg/Rep's CSM >>\nIf you need to tell who triggered this state , use this string. If it's this case itself, this string is \"\"."
                # "#CSM >> Arguments >>\nDeal with the parameter if any"
              }
              frame "API: API2" {
                # "#CSM API Example\nCopy/Rename this case for your own API"
                # "unpack Hex String  to Variant\nif complex parameter is needed."
                n137 = call "CSM - Convert HexStr to Data.vi"("HEX String"=w403) -> ()  [unwired: 7 in, 2 out]
                n138 = disable-structure shown="Disabled" {
                  disable-tunnel: [w407 "API2 Response"] -> w402
                  frame Disabled {
                    # "pack variant to hexstr \nif complex response is needed."
                    # "complex Response"
                    n139 = call "CSM - Convert Data to HexStr.vi"() -> ("HEX String (0-9,A-F)"=w407:string)  [unwired: 9 in]
                  }
                  frame Enabled {
                  }
                }
              }
              frame "---------- Action ----------" {
                # "#CSM \"Category Seperator\"\nDo not put any code in this frame."
                n140 = call <vilib>:"Add State(s) to Queue__JKI_lib_State_Machine.vi"("State(s) in (\"\")"=w412) -> ("States Out"=w411:string)  [unwired: 14 in]
              }
              frame "Action: action1" {
                # "#CSM \"Internal State\"\nThis category is used for holding internal states"
                n141 = call <vilib>:"Add State(s) to Queue__JKI_lib_State_Machine.vi"("State(s) in (\"\")"=w416) -> ("States Out"=w415:string)  [unwired: 14 in]
              }
              frame "Action: action2" {
                # "#CSM \"Internal State\"\nThis category is used for holding internal states"
                n142 = call <vilib>:"Add State(s) to Queue__JKI_lib_State_Machine.vi"("State(s) in (\"\")"=w420) -> ("States Out"=w419:string)  [unwired: 14 in]
              }
            }
          }
          n143 = flat-sequence {
            tunnel: w89 -> [w102]
            tunnel: [w101] -> w86
            tunnel: w84 -> [w100]
            tunnel: w86 -> [w106]
            tunnel: [w105] -> w85
            frame #0 {
              n144 = call "CSM - Send Message and Wait for Reply.vi"("Response Timeout (-2 Using Global Settings)"=60000, "Target Module"=w100, "State"="Macro: Exit") -> ("error out"=w99:errorcluster)  [unwired: 6 in, 2 out]
              n145 = call <vilib>:"Clear Errors.vi"("error in (no error)"=w99) -> ("error out"=w98:errorcluster)  [unwired: 5 in, 1 out]
              n146 = Merge Errors(w102, w98) -> (w101:errorcluster)
            }
            frame #1 {
              n147 = call "CSM - Drop Broadcast Registry.vi"() -> ("error out"=w104:errorcluster)  [unwired: 15 in]
              n148 = Merge Errors(w106, w104) -> (w105:errorcluster)
            }
          }
        }
      }
    }
    frame Disabled {
      # "skip test result while test is under development"
      n149 = call <vilib>:"skip.vi"("error in (no error)"=w421, "TestCase in"=w424) -> ("error out"=w423:errorcluster, "TestCase out"=w422:refnum<class "testcase-CSMBroadcast.lvclass">)  [unwired: 8 in]
    }
  }
  "error out" <- w4
  "TestCase out" <- w2
